vi "ChassisClose.vi"   [LabVIEW 2014, in "ChassisLib.lvlib"]
uses:
  ChassisLib.lvlib
  ChassisRefs.ctl
  <vilib>/Rock Robotics/WPI/RobotDrive/WPI_RobotDriveGetSetRefNum.vi
  <vilib>/Rock Robotics/WPI/Compressor/WPI_CompressorGetSetRefNum.vi
types:
  T1 = typedef "ChassisLib.lvlib/ChassisRefs.ctl" = enum16{"RobotDrive", "Compressor"}
  T2 = typedef "WPI_RobotDriveDevRef.ctl" = cluster{"DevStatus":errorcluster, "Motors[]":T3[], "Square Inputs":bool, "Max Output":dbl}
  T3 = typedef "WPI_MotorControlDeviceRef.ctl" = cluster{"DeviceStatus":errorcluster, "Type":T4, "PWM":cluster{"Controller":T5, "PWM Channel":T6, "DeadBand":T7}, "CAN":cluster{"Device Number":u8, "Control Mode":T8, "Semaphore":T9, "Max Vout":dbl, "TalonSRX Control Mode":T10}, "Invert":bool, "TransformRef":T11, "InvTransformRef":T11}
  T4 = typedef "WPI_MotorControlType.ctl" = enum16{"PWM", "CAN", "CANTalonSRX"}
  T5 = typedef "FPGA_TypedefDigitalModule.ctl" = enum16{"Controller 1"}
  T6 = typedef "FPGA_DIOPWMChannel.ctl" = enum8{"PWM 0", "PWM 1", "PWM 2", "PWM 3", "PWM 4", "PWM 5", "PWM 6", "PWM 7", "PWM 8", "PWM 9", "PWM MXP 0", "PWM MXP 1", "PWM MXP 2", "PWM MXP 3", "PWM MXP 4", "PWM MXP 5", "PWM MXP 6", "PWM MXP 7", "PWM MXP 8", "PWM MXP 9", "Invalid"}
  T7 = typedef "WPI_PWMDeadband.ctl" = cluster{"Name":string, "maxPositivePwm":i32, "minPositivePwm":i32, "centerPwm":i32, "maxNegativePwm":i32, "minNegativePwm":i32, "angularRange":u16}
  T8 = typedef "WPI_CANJaguar_ControlMode.ctl" = enum8{"Percent VBus", "Current", "Speed", "Position", "Voltage"}
  T9 = typedef "Semaphore RefNum" = refnum<k1>
  T10 = typedef "WPI_CANTalonSRX_APIControlMode.ctl" = enum8{"Percent VBus", "Speed", "Position", "Slave", "Unchanged / Invalid"}
  T11 = typedef "WPI_PWMTransform_ConPane.ctl" = refnum<vi>
  T12 = typedef "WPI_CompressorDevRef.ctl" = cluster{"DevStatus":errorcluster, "Pneumatics Control Module":u8}
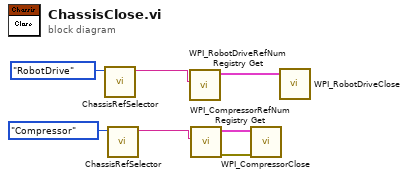
[diagram p0: block diagram]
diagram:
  n1 = call "ChassisRefSelector.vi"("Enum 2"=ChassisRefs."RobotDrive") -> ("String"=w6:string)  [unwired: 10 in]
  n2 = call "ChassisRefSelector.vi"("Enum 2"=ChassisRefs."Compressor") -> ("String"=w1:string)  [unwired: 10 in]
  n3 = call <vilib>:"WPI_RobotDriveRefNum Registry Get.vi"("refnum name"=w6) -> ("RobotDriveDevRef"=w7:T2)  [unwired: 9 in, 1 out]
  n4 = call <vilib>:"WPI_CompressorRefNum Registry Get.vi"("refnum name"=w1) -> ("error out"=w4:errorcluster, "CompressorDevRef"=w3:T12)  [unwired: 9 in]
  n5 = call <vilib>:"WPI_CompressorClose.vi"("error in (no error)"=w4, "CompressorDevRef"=w3) -> ()  [unwired: 9 in, 1 out]
  n6 = call <vilib>:"WPI_RobotDriveClose.vi"("RobotDriveDevRef"=w7) -> ()  [unwired: 10 in, 1 out]
